vi "get_angles.vi"(8 "error in (no error)":errorcluster, 11 "GenericTrajectory in":refnum<class "TrajectoryDL091126GenericVoxel.lvclass">) -> (0 "error out":errorcluster, 1 "current tilting angle":dbl[unit], 2 "current rotation angle":dbl[unit], 3 "GenericTrajectory out":refnum<class "TrajectoryDL091126GenericVoxel.lvclass">)   [LabVIEW 2010, in "TrajectoryDL091126GenericVoxel.lvclass"]
uses:
  TrajectoryDL091126GenericVoxel.lvclass
  TrajectoryDL091126GenericVoxel.lvclass/TrajectoryDL091126GenericVoxel.ctl
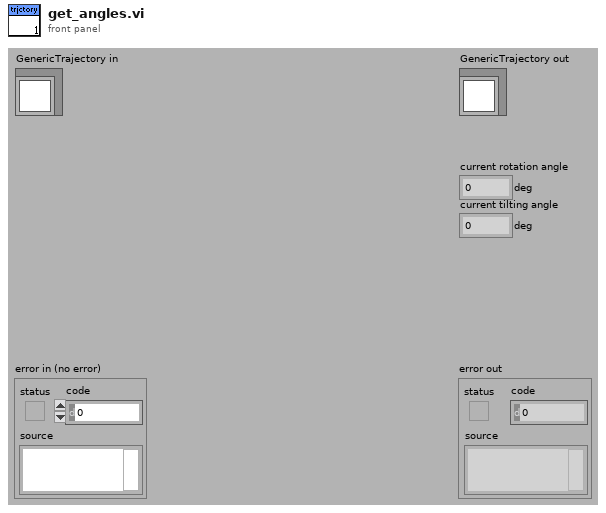
[diagram p1: front panel]
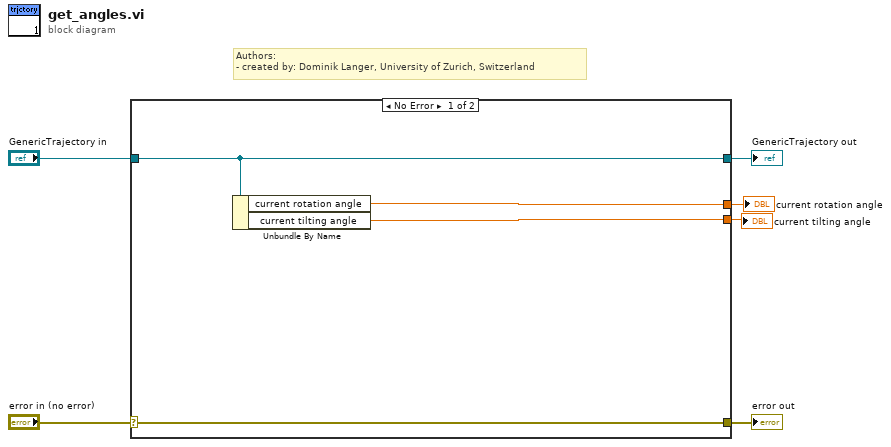
[diagram p0: block diagram]
diagram:
  # "Authors: \n- created by: Dominik Langer, University of Zurich, Switzerland"
  n1 = case shown="No Error" "error in (no error)" {
    selector: "error in (no error)" -> [w10 w12]
    tunnel: [w10 w12] -> w5
    tunnel: [w9 w11] -> w3
    tunnel: "GenericTrajectory in" -> [w9 w11]
    tunnel: [w8 _] -> w2
    tunnel: [w7 _] -> w1
    frame No Error {
      n2 = Unbundle By Name(w9) -> ("current rotation angle"=w8:dbl[unit], "current tilting angle"=w7:dbl[unit])
    }
    frame Error {
    }
  }
  "error out" <- w5
  "GenericTrajectory out" <- w3
  "current rotation angle" <- w2
  "current tilting angle" <- w1
